vi "setupSimulator.vi"(8 "error in (no error)":errorcluster, 11 "IInstance in":refnum<class "IInstance.lvclass">) -> (0 "error out":errorcluster, 3 "IInstance out":refnum<class "IInstance.lvclass">)   [LabVIEW 2022 SP3, in "openDAQ.lvlib" / "daqUtils.lvlib"]
uses:
  <instrlib>/openDAQ/Public/Classes/daqUtils/daqUtils.lvlib
  <instrlib>/openDAQ/Public/Classes/IInstance/IInstance.lvclass
  C:/Program Files (x86)/National Instruments/LabVIEW 2022/instr.lib/openDAQ/Public/Classes/IDevice/IDevice.lvclass
  <instrlib>/openDAQ/Public/Classes/IPropertyObject/Polymorphic/setPropertyValue/setPropertyStringValue.vi
  <instrlib>/openDAQ/Public/Classes/IInstanceBuilder/IInstanceBuilder.lvclass
  <instrlib>/openDAQ/Public/Classes/IPropertyObject/IPropertyObject.lvclass
  <instrlib>/openDAQ/Public/Classes/IDevice/IDevice.lvclass
  <instrlib>/openDAQ/Public/Classes/IServer/IServer.lvclass
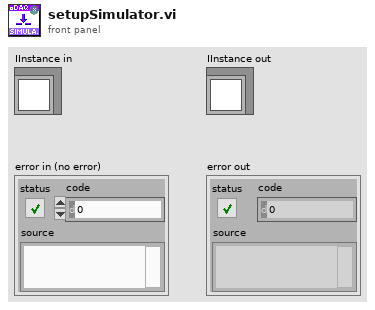
[diagram p1: front panel]
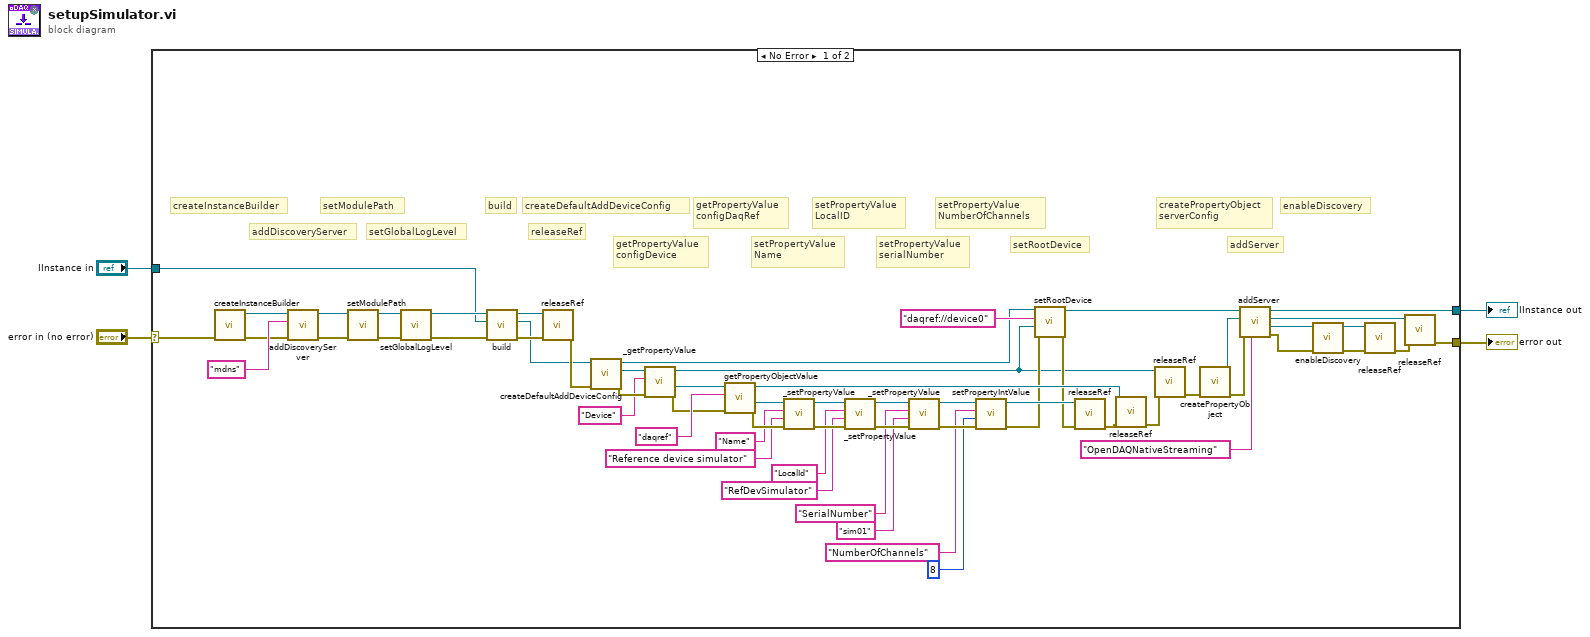
[diagram p0: block diagram]
diagram:
  n1 = case shown="No Error" "error in (no error)" {
    selector: "error in (no error)" -> [w51 w65]
    tunnel: "IInstance in" -> [w52 w64]
    tunnel: [w14 w64] -> w1
    tunnel: [w13 w65] -> w2
    frame No Error {
      # "enableDiscovery"
      # "addServer"
      # "createPropertyObject\nserverConfig"
      # "setRootDevice"
      # "setPropertyValue\nNumberOfChannels"
      # "setPropertyValue\nserialNumber"
      # "setPropertyValue\nLocalID"
      # "setPropertyValue\nName"
      # "getPropertyValue\nconfigDaqRef"
      # "getPropertyValue\nconfigDevice"
      # "createDefaultAddDeviceConfig"
      # "releaseRef"
      # "build"
      # "setGlobalLogLevel"
      # "setModulePath"
      # "addDiscoveryServer"
      # "createInstanceBuilder"
      n2 = call <instrlib>:"createInstanceBuilder.vi"("error in (no error)"=w51) -> ("error out"=w54:errorcluster, "IInstanceBuilder out"=w53:refnum<class "IInstanceBuilder.lvclass">)  [unwired: 9 in]
      n3 = call <instrlib>:"addDiscoveryServer.vi"("error in (no error)"=w54, "DiscoveryServer"="mdns" ("String"), "IInstanceBuilder in"=w53) -> ("error out"=w62:errorcluster, "IInstanceBuilder out"=w50:refnum<class "IInstanceBuilder.lvclass">)  [unwired: 7 in]
      n4 = call <instrlib>:"setModulePath.vi"("error in (no error)"=w62, "IInstanceBuilder in"=w50) -> ("error out"=w57:errorcluster, "IInstanceBuilder out"=w56:refnum<class "IInstanceBuilder.lvclass">)  [unwired: 8 in]
      n5 = call <instrlib>:"setGlobalLogLevel.vi"("error in (no error)"=w57, "IInstanceBuilder in"=w56) -> ("error out"=w59:errorcluster, "IInstanceBuilder out"=w58:refnum<class "IInstanceBuilder.lvclass">)  [unwired: 8 in]
      n6 = call <instrlib>:"build.vi"("error in (no error)"=w59, "Instance in"=w52, "IInstanceBuilder in"=w58) -> ("error out"=w61:errorcluster, "Instance out"=w21:refnum<class "IInstance.lvclass">, "IInstanceBuilder out"=w60:refnum<class "IInstanceBuilder.lvclass">)  [unwired: 6 in]
      n7 = call-dynamic "releaseRef.vi"("error in (no error)"=w61, "IBaseObject in"=w60) -> ("error out"=w49:errorcluster)  [unwired: 9 in]
      n8 = call <instrlib>:"createDefaultAddDeviceConfig.vi"("error in (no error)"=w49, "IDevice in"=w21) -> ("error out"=w63:errorcluster, "Config out"=w46:refnum<class "IPropertyObject.lvclass">, "IDevice out"=w10:refnum<class "IInstance.lvclass">)  [unwired: 7 in]
      n9 = call-poly <instrlib>:"_getPropertyValue.vi"("error in (no error)"=w63, "Property Name in"="Device" ("String"), "IPropertyObject in"=w46) -> ("error out"=w43:errorcluster, "Value out"=w44:refnum<class "IPropertyObject.lvclass">, "IPropertyObject out"=w22:refnum<class "IPropertyObject.lvclass">)  [unwired: 5 in, 1 out]
      n10 = call <instrlib>:"getPropertyObjectValue.vi"("error in (no error)"=w43, "Property Name in"="daqref" ("String"), "IPropertyObject in"=w44) -> ("error out"=w41:errorcluster, "Value out"=w42:refnum<class "IPropertyObject.lvclass">, "IPropertyObject out"=w48:refnum<class "IPropertyObject.lvclass">)  [unwired: 5 in, 1 out]
      n11 = call-poly <instrlib>:"_setPropertyValue.vi"("error in (no error)"=w41, "Property Value in"="Reference device simulator" ("String"), "Property Name in"="Name" ("String"), "IPropertyObject in"=w42) -> ("error out"=w37:errorcluster, "IPropertyObject out"=w38:refnum<class "IPropertyObject.lvclass">)  [unwired: 4 in, 2 out]
      n12 = call-poly <instrlib>:"_setPropertyValue.vi"("error in (no error)"=w37, "Property Value in"="RefDevSimulator" ("String"), "Property Name in"="LocalId" ("String"), "IPropertyObject in"=w38) -> ("error out"=w33:errorcluster, "IPropertyObject out"=w34:refnum<class "IPropertyObject.lvclass">)  [unwired: 4 in, 2 out]
      n13 = call-poly <instrlib>:"_setPropertyValue.vi"("error in (no error)"=w33, "Property Value in"="sim01" ("String"), "Property Name in"="SerialNumber" ("String"), "IPropertyObject in"=w34) -> ("error out"=w29:errorcluster, "IPropertyObject out"=w30:refnum<class "IPropertyObject.lvclass">)  [unwired: 4 in, 2 out]
      n14 = call <instrlib>:"setPropertyIntValue.vi"("error in (no error)"=w29, "Property Value in"=8 ("String"), "Property Name in"="NumberOfChannels" ("String"), "IPropertyObject in"=w30) -> ("error out"=w25:errorcluster, "IPropertyObject out"=w28:refnum<class "IPropertyObject.lvclass">)  [unwired: 4 in, 2 out]
      n15 = call <instrlib>:"setRootDevice.vi"("error in (no error)"=w25, "Config in"=w22, "Connection String in"="daqref://device0" ("String"), "IInstance in"=w10) -> ("error out"=w23:errorcluster, "IInstance out"=w19:refnum<class "IInstance.lvclass">)  [unwired: 4 in, 2 out]
      n16 = call-dynamic "releaseRef.vi"("error in (no error)"=w23, "IBaseObject in"=w28) -> ("error out"=w11:errorcluster)  [unwired: 9 in]
      n17 = call-dynamic "releaseRef.vi"("error in (no error)"=w11, "IBaseObject in"=w48) -> ("error out"=w12:errorcluster)  [unwired: 9 in]
      n18 = call-dynamic "releaseRef.vi"("error in (no error)"=w12, "IBaseObject in"=w22) -> ("error out"=w9:errorcluster)  [unwired: 9 in]
      n19 = call <instrlib>:"createPropertyObject.vi"("error in (no error)"=w9) -> ("error out"=w20:errorcluster, "IPropertyObject out"=w18:refnum<class "IPropertyObject.lvclass">)  [unwired: 9 in]
      n20 = call <instrlib>:"addServer.vi"("TypeString in"="OpenDAQNativeStreaming" ("String"), "error in (no error)"=w20, "ServerConfig in"=w18, "IDevice in"=w19) -> ("error out"=w6:errorcluster, "Server out"=w8:refnum<class "IServer.lvclass">, "ServerConfig out"=w15:refnum<class "IPropertyObject.lvclass">, "IDevice out"=w14:refnum<class "IInstance.lvclass">)  [unwired: 4 in]
      n21 = call <instrlib>:"enableDiscovery.vi"("error in (no error)"=w6, "IServer in"=w8) -> ("error out"=w5:errorcluster, "IServer out"=w7:refnum<class "IServer.lvclass">)  [unwired: 8 in]
      n22 = call-dynamic "releaseRef.vi"("error in (no error)"=w5, "IBaseObject in"=w7) -> ("error out"=w16:errorcluster)  [unwired: 9 in]
      n23 = call-dynamic "releaseRef.vi"("error in (no error)"=w16, "IBaseObject in"=w15) -> ("error out"=w13:errorcluster)  [unwired: 9 in]
    }
    frame Error {
    }
  }
  "IInstance out" <- w1
  "error out" <- w2
